vi "Is Club.vi"(7 "File Path":path=path "C:/PokerSS/7 Club.png", 8 "error in":errorcluster, 11 "ROI Descriptor (Club Match)":T2={"Global Rectangle"=[530, 711, 555, 739], "Contours"=[{"ID"=enum."External", "Type"=12, "Coordinates"=[530, 711, 555, 739, 0]}]} {"Contours"."Type" items=["No Selection", "Point", "Line", "Rectangle", "Oval", "Polygon", "Freehand Region", "Annulus", "Unused2", "Unused3", "Broken Line", "Freehand Line", "Rotated Rectangle"]}) -> (0 "error out":errorcluster, 2 "Suit":T1(ring), 3 "IS Club":bool)   [LabVIEW 2015]
uses:
  <vilib>/vision/NI_Vision_Development_Module.lvlib
panel:
  out "Image Out":T3(plugin-control)
  out "Matches (Club Match)":T4(array[cluster]) {"Bounding Box"."y" format="%.2f"; "Bounding Box"."x" format="%.2f"; "Position"."y" format="%.2f"; "Position"."x" format="%.2f"; "Score" format="%.2f"; "Scale" format="%.2f"; "Angle" format="%.2f"}
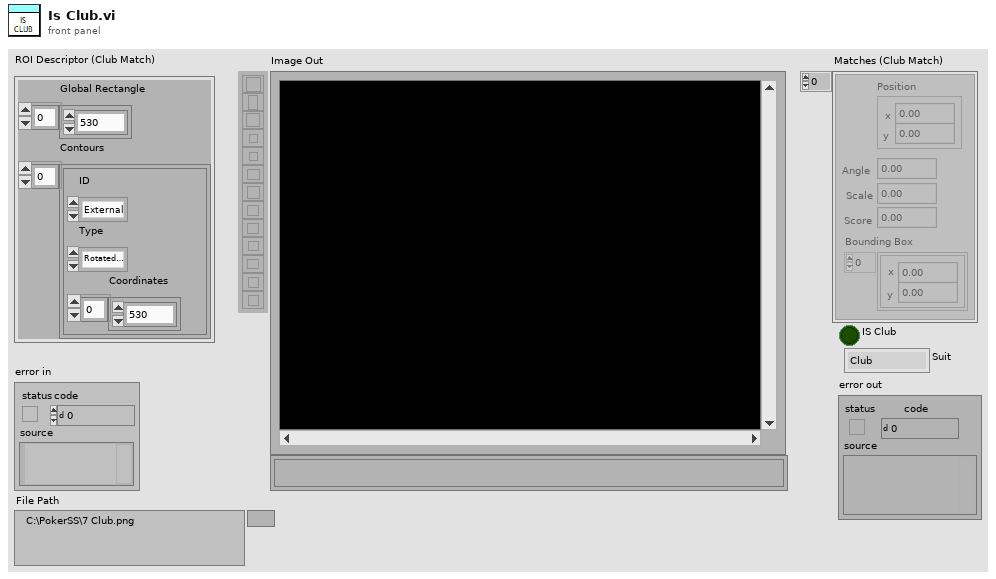
[diagram p1: front panel]
types:
  T1 = enum16{"Club", "Diamond", "Heart", "Spade", "Unknown"}
  T2 = cluster{"Global Rectangle":i32[], "Contours":cluster{"ID":enum32{"External", "Internal"}, "Type":u32, "Coordinates":i32[]}[]}
  T3 = typedef "IMAQ Image.ctl" = refnum<image>
  T4 = cluster{"Position":cluster{"x":sgl, "y":sgl}, "Angle":sgl, "Scale":sgl, "Score":sgl, "Bounding Box":cluster{"x":sgl, "y":sgl}[]}[]
  T5 = cluster{"Number of Matches Requested":i32, "Minimum Match Score":sgl, "Angle Ranges":cluster{"Start Angle":sgl, "End Angle":sgl}[]}
  T6 = typedef "Image Type" = u32
  T7 = cluster{"Position":cluster{"x":sgl, "y":sgl}, "Angle":sgl, "Scale":sgl, "Score":sgl, "Bounding Box":cluster{"x":sgl, "y":sgl}[]}
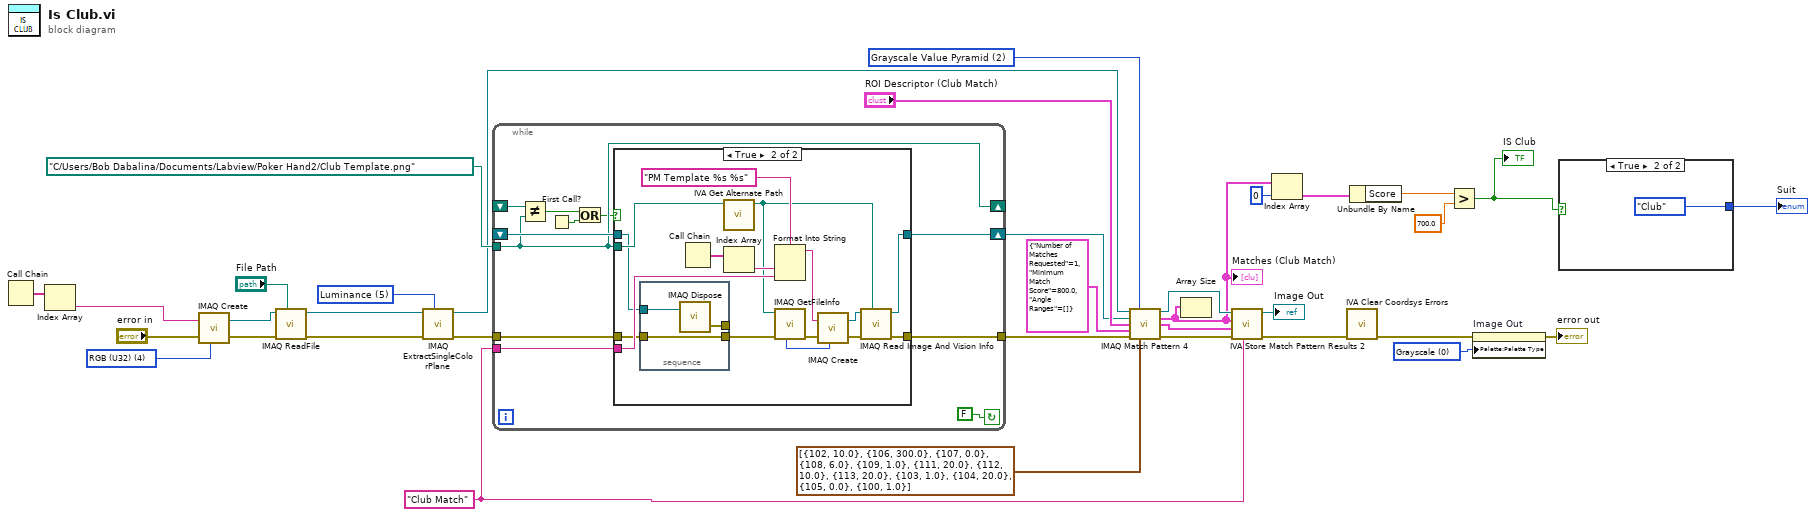
[diagram p0: block diagram]
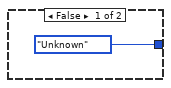
[diagram p2: hidden frame]
diagram:
  w9 = u32 0 items=["Grayscale", "Binary", "Gradient", "Rainbow", "Temperature", "User Defined", "Binary 16 Bit", "Gradient 16 Bit", "Rainbow 16 Bit", "Temperature 16 Bit", "User Defined 16 Bit"] ("Palette Type")
  w21 = 2 items=["All", "Low Discrepancy Sampling", "Grayscale Value Pyramid", "Gradients Pyramid"] ("Algorithm")
  w18 = "Club Match" ("Step Name")
  w28 = 5 items=["Red", "Green", "Blue", "Hue", "Saturation", "Luminance", "Value", "Intensity"] ("Color Plane")
  w29 = T6 4 items=["Grayscale (U8)", "Grayscale (I16)", "Grayscale (SGL)", "Complex (CSG)", "RGB (U32)", "HSL (U32)", "RGB (U64)", "Grayscale (U16)"] ("Image Type")
  n1 = Call Chain() -> (call chain=w31:string[])
  n2 = Index Array(array=w31) -> (element=w30:string)  [unwired: 1 in]
  n3 = call "IMAQ Create"("Image Name"=w30, "Image Type"=w29, "error in (no error)"="error in") -> ("New Image"=w34:T3, "error out"=w33:errorcluster)  [unwired: 1 in, 1 out]
  n4 = call "IMAQ ReadFile"("File Path"="File Path", "error in (no error)"=w33, "Image"=w34) -> ("error out"=w35:errorcluster, "Image Out"=w27:T3)  [unwired: 2 in, 5 out]
  n5 = call "IMAQ ExtractSingleColorPlane"("Color Plane"=w28, "error in (no error)"=w35, "Image Src"=w27) -> ("error out"=w26:errorcluster, "Image Dst Out"=w24:T3)  [unwired: 1 in, 6 out]
  n6 = while {
    shift-right: [w46] -> w16
    shift-left: _ -> [w45]
    tunnel: [w43] -> w15
    tunnel: w26 -> [w42]
    tunnel: path "C:/Users/Bob Dabalina/Documents/Labview/Poker Hand2/Club Template.png" ("Template File Path") -> [w39]
    tunnel: w18 -> [w41]
    shift-right: [w39] -> _
    shift-left: _ -> [w40]
    stop <- FALSE continue-if-true
    n7 = Not Equal?(x=w40, y=w39) -> (x != y?=w37:bool)
    n8 = First Call?() -> (First Call?: T/F=w38:bool)
    n9 = Or(x=w37, y=w38) -> (x .or. y?=w36:bool)
    n10 = case shown="True" w36 {
      tunnel: [w48 w62] -> w46
      tunnel: w45 -> [w48 w54]
      tunnel: [w47 w59] -> w43
      tunnel: w42 -> [w47 w53]
      tunnel: w39 -> [_ w55]
      tunnel: w41 -> [_ w56]
      frame False {
      }
      frame True {
        n11 = stacked-sequence {
          tunnel: w54 -> [w67]
          tunnel: w53 -> [w66]
          tunnel: [w66] -> w49
          tunnel: [w65] -> _
          frame #0 {
            n12 = call "IMAQ Dispose"("Image"=w67) -> ("error out"=w65:errorcluster)  [unwired: 2 in, 3 out]
          }
        }
        n13 = Call Chain() -> (call chain=w58:string[])
        n14 = call <vilib>:"IVA Get Alternate Path.vi"("Path In"=w55) -> ("Path Out"=w51:path)  [unwired: 10 out]
        n15 = Index Array(array=w58) -> (element=w57:string)  [unwired: 1 in]
        n16 = Format Into String(format string="PM Template %s %s" ("Image Name"), w57, w56) -> (resulting string=w64:string)  [unwired: 2 in, 1 out]
        n17 = call "IMAQ GetFileInfo"("error in (no error)"=w49, "File Path"=w51) -> ("error out"=w50:errorcluster, "Image Type"=w52:T6)  [unwired: 3 in, 5 out]
        n18 = call "IMAQ Create"("Image Name"=w64, "Image Type"=w52, "error in (no error)"=w50) -> ("New Image"=w61:T3, "error out"=w60:errorcluster)  [unwired: 1 in, 1 out]
        n19 = call "IMAQ Read Image And Vision Info"("File Path"=w51, "error in (no error)"=w60, "Image"=w61) -> ("error out"=w59:errorcluster, "Image Out"=w62:T3)  [unwired: 1 in, 6 out]
      }
    }
  }
  n20 = call "IMAQ Match Pattern 4"("Image"=w24, "Algorithm"=w21, "Template Image"=w16, "ROI Descriptor"="ROI Descriptor (Club Match)", "Parameters"=T5 {"Number of Matches Requested"=1, "Minimum Match Score"=800.0, "Angle Ranges"=[]}, "error in (no error)"=w15, "Advanced Options"=cluster{"Item":u16, "Value":dbl}[] [{"Item"=102, "Value"=10.0}, {"Item"=106, "Value"=300.0}, {"Item"=107, "Value"=0.0}, {"Item"=108, "Value"=6.0}, {"Item"=109, "Value"=1.0}, {"Item"=111, "Value"=20.0}, {"Item"=112, "Value"=10.0}, {"Item"=113, "Value"=20.0}, {"Item"=103, "Value"=1.0}, {"Item"=104, "Value"=20.0}, {"Item"=105, "Value"=0.0}, {"Item"=100, "Value"=1.0}]) -> ("Image (duplicate)"=w22:T3, "Matches (pixel)"=w7:T4, "Matches (real-world)"=w17:T4, "error out"=w23:errorcluster)  [unwired: 4 in, 1 out]
  "Matches (Club Match)" <- w7
  n21 = Array Size(array=w7) -> ()  [unwired: 1 out]
  n22 = call <vilib>:"IVA Store Match Pattern Results 2.vi"("Step Name"=w18, "error in (no error)"=w23, "Matches (real-world)"=w17, "Matches (pixel)"=w7, "Image in"=w22) -> ("error out"=w14:errorcluster, "Image dup"=→"Image Out":T3)  [unwired: 1 in, 4 out]
  n23 = Index Array(array=w7, index=0) -> (element=w5:T7)
  n24 = call <vilib>:"IVA Clear Coordsys Errors.vi"("error in (no error)"=w14) -> ("error out"=w13:errorcluster)  [unwired: 10 in]
  n25 = Unbundle By Name(w5) -> ("Score"=w3:sgl)
  n26 = Greater?(x=w3, y=700.0) -> (0:w2:bool)
  "IS Club" <- w2
  n27 = property on="Image Out" class="ImageControl"(error in=w13, "Palette:Palette Type"=w9) -> (error out=→"error out":errorcluster)  [unwired: 1 in, 1 out]
  n28 = case shown="True" w2 {
    tunnel: [T1."Unknown" T1."Club"] -> w1
    frame False {
    }
    frame True {
    }
  }
  "Suit" <- w1
